vi "Generate Signals.vi"(5 "Sample Rate":dbl=10000000.0 format="%#_13p", 7 "SPI Configuration":T1={"CLK Frequency (Hz)"=250000, "CPOL"=FALSE, "CPHA"=FALSE, "CS Channel"="", "CLK Channel"="", "MOSI Channel"="", "MISO Channel"="", "Active CS"=FALSE, "Dig In Task"="", "Dig Out Task"=""} {"CLK Frequency (Hz)" format="%#.6p"}, 8 "Error In":errorcluster, 11 "MOSI Data":u8[](array[numeric]) format="%x") -> (0 "Error Out":errorcluster, 3 "Signals":digitalwaveform(waveform)={"t0"=timestamp(0 s since 1904-01-01), "dt"=0.0, "Y"={"transitions"=[], "data"=[]}, "error"={"status"=FALSE, "code"=37421928, "source"=""}})   [LabVIEW 2016, in "SPIVI.lvlib"]
uses:
  SPIVI.lvlib
  Typedefs/SPI Configuration.ctl
  <userlib>/SPI Digital Waveform/_Typedefs/Timing-ns.ctl
  <userlib>/SPI Digital Waveform/_Typedefs/Bus config.ctl
  <userlib>/SPI Digital Waveform/_Polymorphics/Init-Preallocate-fmt0.vi
  <userlib>/SPI Digital Waveform/_Polymorphics/Close-fmt0.vi
  <vilib>/Waveform/DWDTOps.llb/DWDT Digital Signal Subset.vi
  <userlib>/SPI Digital Waveform/SDW.lvlib
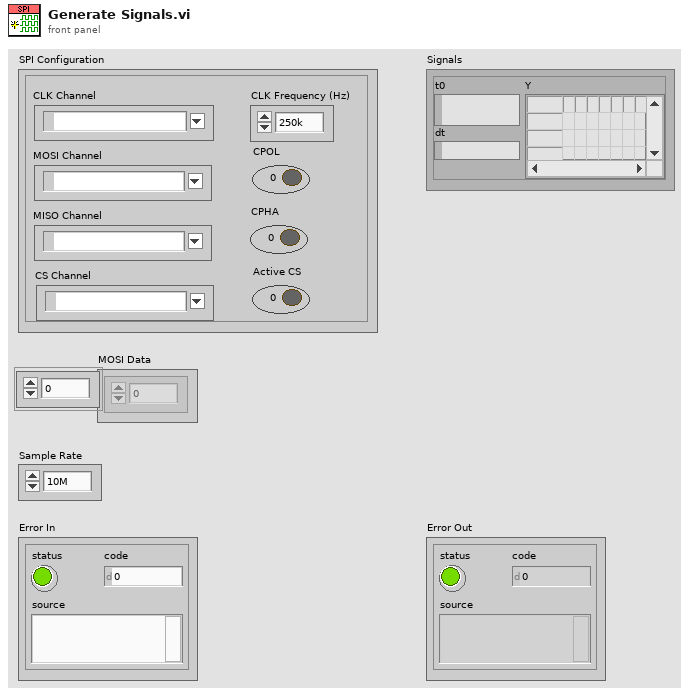
[diagram p1: front panel]
types:
  T1 = typedef "SPIVI.lvlib/SPI Configuration.ctl" = cluster{"CLK Frequency (Hz)":u32, "CPOL":bool, "CPHA":bool, "CS Channel":tag, "CLK Channel":tag, "MOSI Channel":tag, "MISO Channel":tag, "Active CS":bool, "Dig In Task":refnum<k21>, "Dig Out Task":refnum<k21>}
  T2 = typedef "SDW.lvlib/Bus config.ctl" = cluster{"CPOL":bool, "CS active state":bool, "# of slaves":u8}
  T3 = typedef "SDW.lvlib/Timing-ns.ctl" = cluster{"MOSI Setup":dbl, "SCLK Freq":dbl, "SCLK Hold":dbl, "CS Lead":dbl, "CS Trail":dbl, "CS Idle":dbl}
  T4 = typedef "SDW.lvlib/Waveform info-fmt0.ctl" = cluster{"Data":u8[][], "Last sample":u8[], "Preallocated":bool, "Sample offset":u64, "Compare offset":u64, "Compare locations":u64[], "SPI timing (ticks)":T5, "CPOL":bool, "CS active":bool}
  T5 = typedef "SDW.lvlib/Timing-ticks-fmt0.ctl" = cluster{"Idle":i32, "CSa-SU":i32, "SU-SCLKa":i32, "SCLKa-SCLKd":i32, "SCLKd-SU":i32, "SCLKd-CSd":i32}
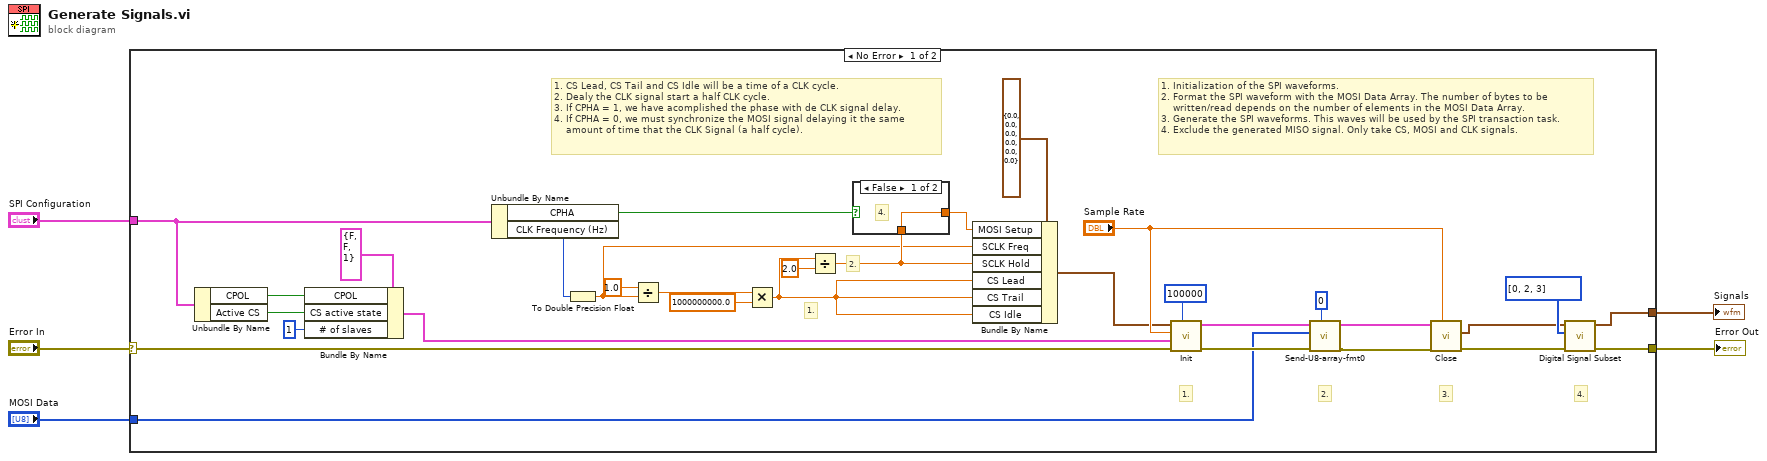
[diagram p0: block diagram]
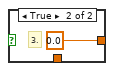
[diagram p2: hidden frame]
diagram:
  n1 = case shown="No Error" "Error In" {
    selector: "Error In" -> [w9 w40]
    tunnel: "SPI Configuration" -> [w10 _]
    tunnel: "MOSI Data" -> [w8 _]
    tunnel: [w7 _] -> w2
    tunnel: [w6 w40] -> w1
    frame No Error {
      # "1. Initialization of the SPI waveforms.\n2. Format the SPI waveform with the MOSI Data Array. The number of bytes to be\n    written/read depends on the number of elements in the MOSI Data Array.\n3. Generate the SPI waveforms. This waves will be used by the SPI transaction task.\n4. Exclude the generated MISO signal. Only take CS, MOSI and CLK signals."
      # "3."
      # "2."
      # "1."
      # "4."
      # "2."
      # "1."
      # "1. CS Lead, CS Tail and CS Idle will be a time of a CLK cycle.\n2. Dealy the CLK signal start a half CLK cycle.\n3. If CPHA = 1, we have acomplished the phase with de CLK signal delay.\n4. If CPHA = 0, we must synchronize the MOSI signal delaying it the same\n    amount of time that the CLK Signal (a half cycle)."
      n2 = Unbundle By Name(w10) -> ("CPOL"=w29:bool, "Active CS"=w30:bool)
      n3 = Bundle By Name(cluster=T2 {"CPOL"=FALSE, "CS active state"=FALSE, "# of slaves"=1} ("Bus configuration"), "CPOL"=w29, "CS active state"=w30, "# of slaves"=u8 1) -> (w24:T2)
      n4 = Unbundle By Name(w10) -> ("CPHA"=w31:bool, "CLK Frequency (Hz)"=w32:u32)
      n5 = To Double Precision Float(number=w32) -> (double precision float=w16:dbl)
      n6 = Divide(x=1.0, y=w16) -> (x/y=w13:dbl)
      n7 = Multiply(x=w13, y=1000000000.0) -> (x*y=w17:dbl)
      n8 = Divide(x=w17, y=2.0) -> (x/y=w20:dbl)
      n9 = case shown="False" w31 {
        tunnel: [w38 0.0] -> w19
        tunnel: w20 -> [w38 _]
        frame False {
          # "4."
        }
        frame True {
          # "3."
        }
      }
      n10 = Bundle By Name(cluster=T3 {"MOSI Setup"=0.0, "SCLK Freq"=0.0, "SCLK Hold"=0.0, "CS Lead"=0.0, "CS Trail"=0.0, "CS Idle"=0.0} ("SPI timing (ns)"), "MOSI Setup"=w19, "SCLK Freq"=w16, "SCLK Hold"=w20, "CS Lead"=w17, "CS Trail"=w17, "CS Idle"=w17) -> (w23:T3)
      n11 = call-poly <userlib>:"Init.vi"("Samples to allocate"=100000, "error in (no error)"=w9, "Bus configuration"=w24, "Sample rate"="Sample Rate", "SPI timing (ns)"=w23) -> ("error out"=w35:errorcluster, "SPI waveform info"=w33:T4)  [unwired: 4 in, 1 out]
      n12 = call "Send-U8-array-fmt0.vi"("Slave address"=u8 0, "error in (no error)"=w35, "MOSI Data"=w8, "SPI waveform info"=w33) -> ("error out"=w36:errorcluster, "SPI waveform info out"=w34:T4)  [unwired: 6 in]
      n13 = call-poly <userlib>:"Close.vi"("Sample rate"="Sample Rate", "error in (no error)"=w36, "SPI waveform info"=w34) -> ("error out"=w26:errorcluster, "Dig waveform out"=w25:digitalwaveform)  [unwired: 6 in, 1 out]
      n14 = call-poly <vilib>:"Digital Signal Subset.vi"("error in (no error)"=w26, "signals"=i32[] [0, 2, 3], "digital waveform"=w25) -> ("error out"=w6:errorcluster, "digital subset"=w7:digitalwaveform)  [unwired: 7 in]
    }
    frame Error {
    }
  }
  "Signals" <- w2
  "Error Out" <- w1
